vi "usbpt104ChannelSetting.vi"(8 "error in (no error)":errorcluster, 10 "Channel Settings":T1={"CH1 # Wires"=4, "CH1 Measurement Type"=1, "CH2 # Wires"=2, "CH2 Measurement Type"=0, "CH3 # Wires"=2, "CH3 Measurement Type"=0, "CH4 # Wires"=2, "CH4 Measurement Type"=0} {"CH4 Measurement Type" items=["OFF", "PT100", "PT1000", "Resistance to 375 Ohms", "Resistance to 10 kOhms", "Differential to 115 mV", "Differential to 2500 mV", "Single-ended to 115 mV", "Single-ended to 2500 mV"]; "CH4 # Wires" items=["2"=2, "3"=3, "4"=4]; "CH3 Measurement Type" items=["OFF", "PT100", "PT1000", "Resistance to 375 Ohms", "Resistance to 10 kOhms", "Differential to 115 mV", "Differential to 2500 mV", "Single-ended to 115 mV", "Single-ended to 2500 mV"]; "CH3 # Wires" items=["2"=2, "3"=3, "4"=4]; "CH2 Measurement Type" items=["OFF", "PT100", "PT1000", "Resistance to 375 Ohms", "Resistance to 10 kOhms", "Differential to 115 mV", "Differential to 2500 mV", "Single-ended to 115 mV", "Single-ended to 2500 mV"]; "CH2 # Wires" items=["2"=2, "3"=3, "4"=4]; "CH1 Measurement Type" items=["OFF", "PT100", "PT1000", "Resistance to 375 Ohms", "Resistance to 10 kOhms", "Differential to 115 mV", "Differential to 2500 mV", "Single-ended to 115 mV", "Single-ended to 2500 mV"]; "CH1 # Wires" items=["2"=2, "3"=3, "4"=4]}, 11 "Handle In":i16) -> (0 "error out":errorcluster, 2 "Channel Enable Array":u8[](array[numeric]), 3 "Handle out":i16)   [LabVIEW 2010]
uses:
  UsbPT104.dll
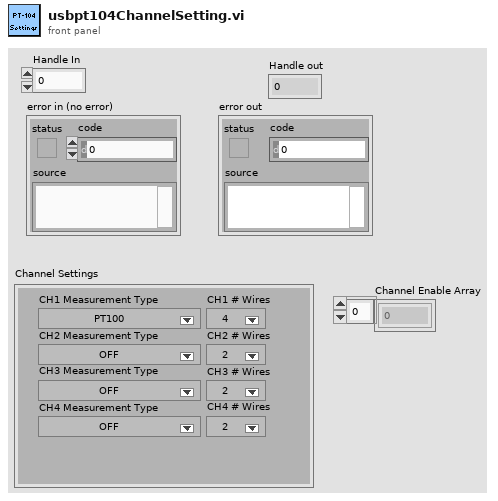
[diagram p1: front panel]
types:
  T1 = cluster{"CH1 # Wires":i16, "CH1 Measurement Type":i32, "CH2 # Wires":i16, "CH2 Measurement Type":i32, "CH3 # Wires":i16, "CH3 Measurement Type":i32, "CH4 # Wires":i16, "CH4 Measurement Type":i32}
  T2 = cluster{"status":bool, "code":u32, "source":string}
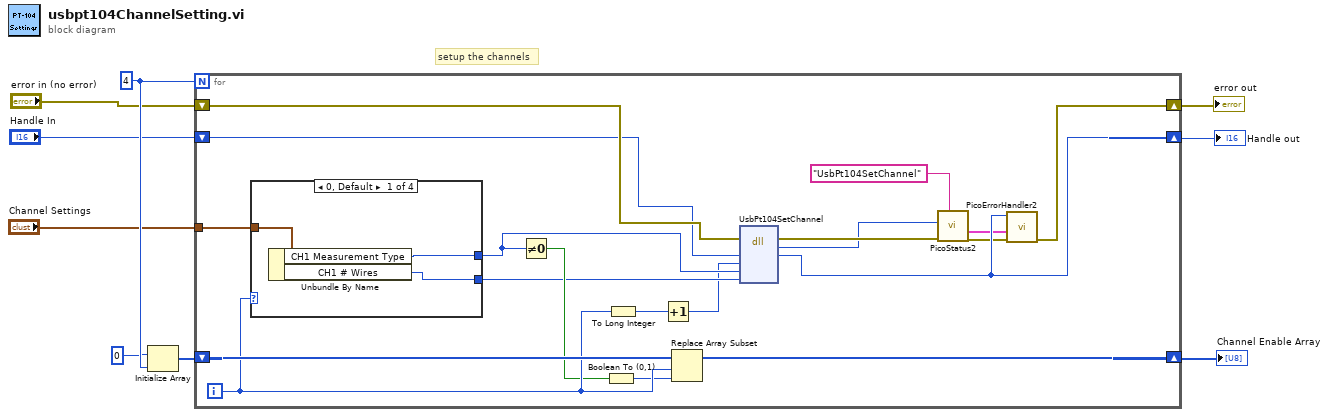
[diagram p0: block diagram]
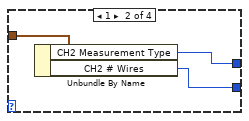
[diagram p2: hidden frame]
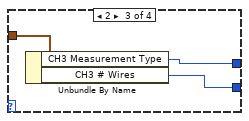
[diagram p3: hidden frame]
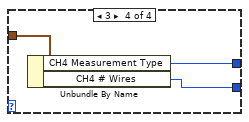
[diagram p4: hidden frame]
diagram:
  w8 = 4
  # "setup the channels"
  n1 = Initialize Array(u8 0 ("element"), w8) -> (w6:u8[])
  n2 = for {
    N: w8 -> [_]
    shift-right: [w28] -> w9
    shift-left: w6 -> [w27]
    shift-right: [w17] -> w5
    shift-left: "Handle In" -> [w23]
    shift-right: [w18] -> w1
    shift-left: "error in (no error)" -> [w24]
    tunnel: "Channel Settings" -> [w22]
    i -> [w26]
    n3 = case shown="0, Default" w26 {
      tunnel: w22 -> [w31 w34 w37 w40]
      tunnel: [w30 w32 w36 w38] -> w20
      tunnel: [w29 w33 w35 w39] -> w19
      frame 0, Default {
        n4 = Unbundle By Name(w31) -> ("CH1 Measurement Type"=w30:i32, "CH1 # Wires"=w29:i16)
      }
      frame 1 {
        n5 = Unbundle By Name(w34) -> ("CH2 Measurement Type"=w32:i32, "CH2 # Wires"=w33:i16)
      }
      frame 2 {
        n6 = Unbundle By Name(w37) -> ("CH3 Measurement Type"=w36:i32, "CH3 # Wires"=w35:i16)
      }
      frame 3 {
        n7 = Unbundle By Name(w40) -> ("CH4 Measurement Type"=w38:i32, "CH4 # Wires"=w39:i16)
      }
    }
    n8 = Not Equal To 0?(x=w20) -> (x != 0?=w21:bool)
    n9 = Boolean To (0,1)(Boolean=w21) -> (0, 1=w25:i16)
    n10 = To Long Integer(number=w26) -> (32bit integer=w16:i32)
    n11 = Increment(x=w16) -> (x+1=w15:i32)
    n12 = Replace Array Subset(array=w27, new element=w25, index=w26) -> (w28:u8[])
    n13 = dll-call lib="UsbPT104.dll" fn="UsbPt104SetChannel"(error in=w24, "handle"=w23, "channel"=w15, "type"=w20, "noOfWires"=w19) -> (error out=w13:errorcluster, "PICO_STATUS"=w10:u32, "handle"=w17:i16)  [unwired: 5 in, 1 out]
    n14 = call "PicoStatus2.vi"("PICO source"="UsbPt104SetChannel" ("source"), "Error in"=w13, "PICO STATUS"=w10) -> ("error out"=w14:errorcluster, "PICO_STATUS out"=w12:T2)  [unwired: 5 in]
    n15 = call "PicoErrorHandler2.vi"("error in (no error)"=w14, "PICO_STATUS in"=w12, "handle In"=w17) -> ("error out"=w18:errorcluster)  [unwired: 8 in]
  }
  "Channel Enable Array" <- w9
  "Handle out" <- w5
  "error out" <- w1
